vi "myRIO_BRig_RT__Case_Exp_State_endBlock.vi"(8 "input_spout":enum16{"Left", "Right"}(ring), 10 "input_dataBlock":u16[][](array[numeric]), 11 "input_dataCurrent":u16[](array[numeric])) -> (2 "output_dataBlock":u16[][](array[numeric]), 3 "output_dataCurrent":u16[](array[numeric]))   [LabVIEW 2014]
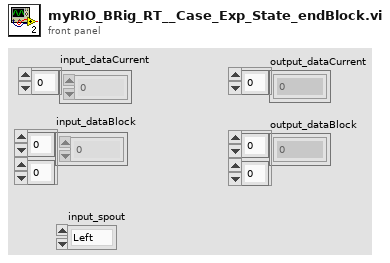
[diagram p1: front panel]
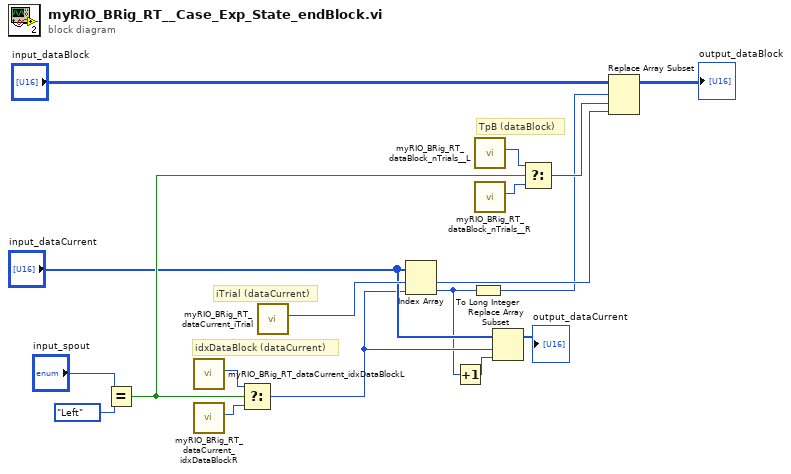
[diagram p0: block diagram]
diagram:
  # "TpB (dataBlock)"
  # "idxDataBlock (dataCurrent)"
  # "iTrial (dataCurrent)"
  n1 = Equal?(x="input_spout", y=enum16{"Left", "Right"}."Left") -> (x = y?=w11:bool)
  n2 = call "myRIO_BRig_RT_dataCurrent_idxDataBlockL.vi"() -> ("output_idxDataBlock__L"=w16:i32)  [unwired: 11 in]
  n3 = call "myRIO_BRig_RT_dataCurrent_idxDataBlockR.vi"() -> ("output_idxDataBlock__R"=w15:i32)  [unwired: 11 in]
  n4 = Select(t=w16, s=w11, f=w15) -> (s? t:f=w4:i32)
  n5 = call "myRIO_BRig_RT_dataCurrent_iTrial.vi"() -> ("output_iTrial"=w14:i32)  [unwired: 11 in]
  n6 = Index Array(array="input_dataCurrent", index #1=w14, index #2=w4) -> (element #1=w8:u16, element #2=w2:u16)
  n7 = Increment(x=w2) -> (x+1=w3:u16)
  n8 = To Long Integer(number=w2) -> (32bit integer=w7:i32)
  n9 = call "myRIO_BRig_RT_dataBlock_nTrials__L.vi"() -> ("output_nTrials__L"=w13:i32)  [unwired: 11 in]
  n10 = call "myRIO_BRig_RT_dataBlock_nTrials__R.vi"() -> ("output_TPB__R"=w12:i32)  [unwired: 11 in]
  n11 = Replace Array Subset(array="input_dataCurrent", new element=w3, index=w4) -> (→"output_dataCurrent":u16[])
  n12 = Select(t=w13, s=w11, f=w12) -> (s? t:f=w9:i32)
  n13 = Replace Array Subset(array="input_dataBlock", new element=w8, index (row)=w7, index (col)=w9) -> (→"output_dataBlock":u16[][])
